vi "shift register.vi"() -> ()   [LabVIEW 2017]
panel:
  out "appended array":i32[](array[numeric])
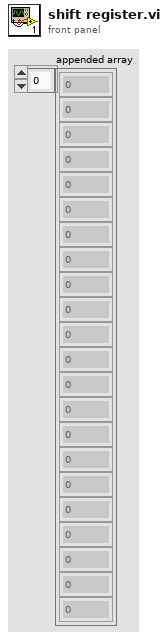
[diagram p1: front panel]
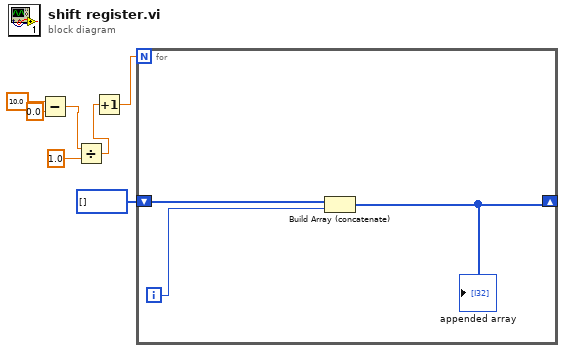
[diagram p0: block diagram]
diagram:
  n1 = Subtract(x=10.0, y=0.0) -> (x-y=w4:dbl)
  n2 = Divide(x=w4, y=1.0) -> (x/y=w2:dbl)
  n3 = Increment(x=w2) -> (x+1=w5:dbl)
  n4 = for {
    N: w5 -> [_]
    shift-right: [w9] -> _
    shift-left: i32[] [] -> [w8]
    i -> [w10]
    n5 = Build Array (concatenate)(w8, w10) -> (w9:i32[])
    "appended array" <- w9
  }
